vi "BASE.SetConfig.vi"(8 "error in (no error)":errorcluster, 10 "config":T1, 11 "BASE in":refnum<class "BASE.lvclass">) -> (0 "error out":errorcluster, 3 "BASE out":refnum<class "BASE.lvclass">)   [LabVIEW 2019, in "BASE.lvlib" / "BASE.lvclass"]
uses:
  BASE.lvclass
  config--cluster.ctl
  BASE.lvclass/BASE.ctl
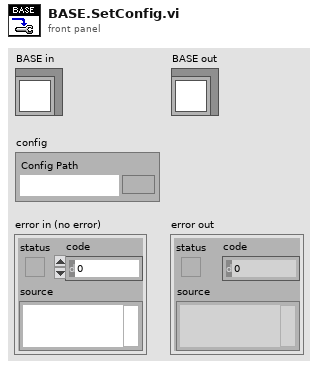
[diagram p1: front panel]
types:
  T1 = typedef "BASE.lvlib/BASE.lvclass/config--cluster.ctl" = cluster{"Config Path":path}
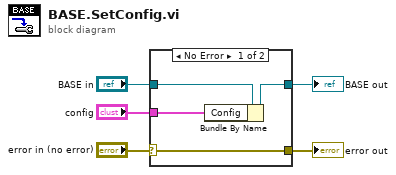
[diagram p0: block diagram]
diagram:
  n1 = case shown="No Error" "error in (no error)" {
    selector: "error in (no error)" -> [w9 w10]
    tunnel: [w9 w10] -> w4
    tunnel: [w7 w11] -> w2
    tunnel: "BASE in" -> [w8 w11]
    tunnel: "config" -> [w6 _]
    frame No Error {
      n2 = Bundle By Name(cluster=w8, "Config"=w6) -> (w7:refnum<class "BASE.lvclass">)
    }
    frame Error {
    }
  }
  "error out" <- w4
  "BASE out" <- w2
